vi "macro_BumplessTransfer.vi"   [LabVIEW 2019, in "Trajectory_Library.lvlib"]
uses:
  Trajectory_Library.lvlib
  SlewRateLimiter_Execute.vi
  Util_GetTime.vi
  SlewRateLimiter_New.vi
  SlewRateLimiter_Reset.vi
  SlewRateLimiter_Calculate.vi
  SlewRateLimiter_SetRate.vi
  VI/Util_GetTime_U32.vi
  VI/Util_GetTime_U64.vi
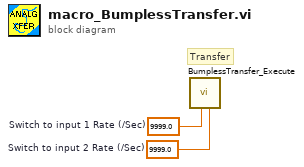
[diagram p0: block diagram]
diagram:
  w1 = 9999.0  # Switch to input 2 Rate (/Sec)
  w2 = 9999.0  # Switch to input 1 Rate (/Sec)
  # "Transfer"
  n1 = call "BumplessTransfer_Execute.vi"("Rate 2"=w1, "Rate 1"=w2) -> ()  [unwired: 9 in, 1 out]
